vi "MAAP3.vi"(0 "Header Comments":string="This is a C(T) experiment being done in Physics 350.\r\nIt records the decay response of an RC circuit where the capacitance is a strong function of temperature.", 9 "Timing control parameters":T2={"N cycles for averaging"=10, "N points per measurment"=1000, "Measurment time interval"=2e-05} {"Measurment time interval" format="%.2e"}, 11 "error in":errorcluster) -> (3 "Proceed":bool=TRUE, 4 "data file path out":path, 6 "Temp Array":dbl[](array[numeric])=[30.0, 40.0, 50.0, 60.0, 70.0, 80.0], 10 "Timing Control Parameters out":T2={"N cycles for averaging"=10, "N points per measurment"=1000, "Measurment time interval"=2e-05} {"Measurment time interval" format="%.2e"}, 14 "Auto Launch Data Viewer at End":bool=TRUE)   [LabVIEW 2016]
doc: "This vi opens a file from the path input and reads a text header then build temp control and time control parameters. These parametars can be modified manually and then an array of temperatures will be created.\n\nMuhannad Alghamdi\nProject 3\nCSUSB Physics 350"
uses:
  typedefs/time_control_params.ctl
  typedefs/temp_control_params.ctl
panel:
  out "error out":errorcluster
  in  "Temp control parameters":T1={"Start Temp"=30.0, "Temp Step"=10.0, "End Temp"=80.0} {"End Temp" format="%.2f"; "Temp Step" format="%.2f"; "Start Temp" format="%.2f"}
  in  "Reload parameters":bool
  in  "Exit":bool
  in  "Create file and proceed":bool
  out "File Header":string="This is a C(T) experiment being done in Physics 350.\r\nIt records the decay response of an RC circuit where the capacitance is a strong function of temperature.\n\n2/16/2017\n12:19 PM\n\nStart temp = 30.000000\nTemp step = 10.000000\nEnd temp = 80.000000\nNum temps = 6\nNum avg cycles = 10\nNum points per meas = 1000\nMeas time interval = 2.000000E-5\n\n<data below>\n\n"
  out "N temps":i32=6
  in  "Auto Launch Data Viewer at End":bool=TRUE
  # "P350 C(T) Experimental Initialization"
  # "Muhanad Alghamdi\nProject 3\nCSUSB Physics 350"
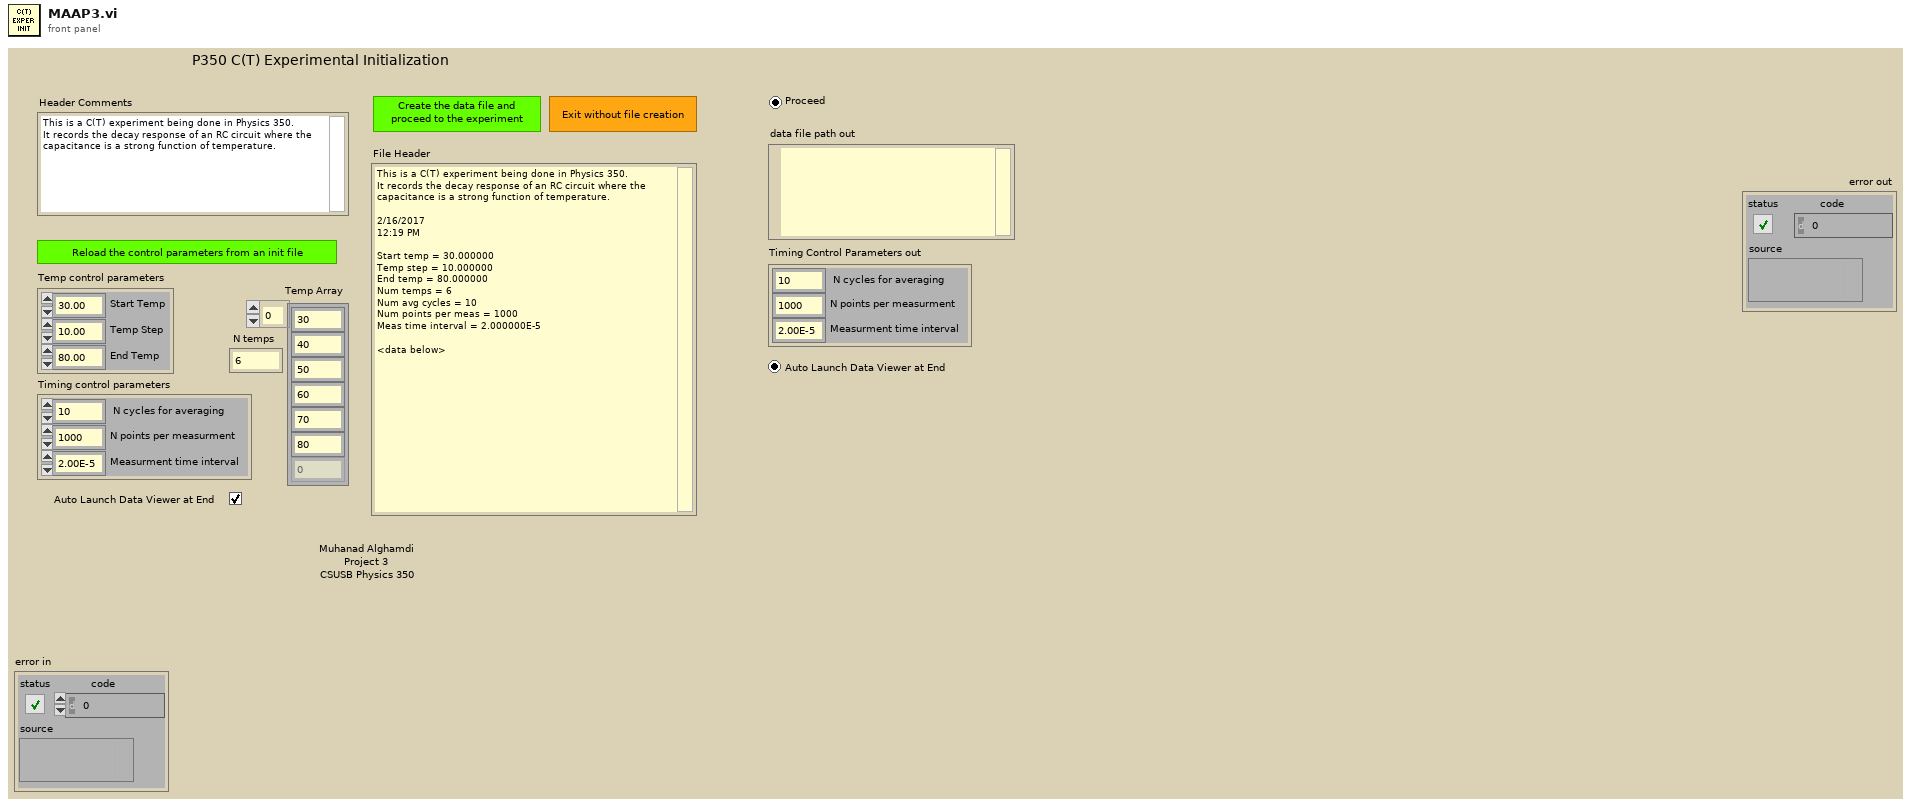
[diagram p1: front panel]
types:
  T1 = typedef "temp_control_params.ctl" = cluster{"Start Temp":dbl, "Temp Step":dbl, "End Temp":dbl}
  T2 = typedef "time_control_params.ctl" = cluster{"N cycles for averaging":i32, "N points per measurment":i32, "Measurment time interval":dbl}
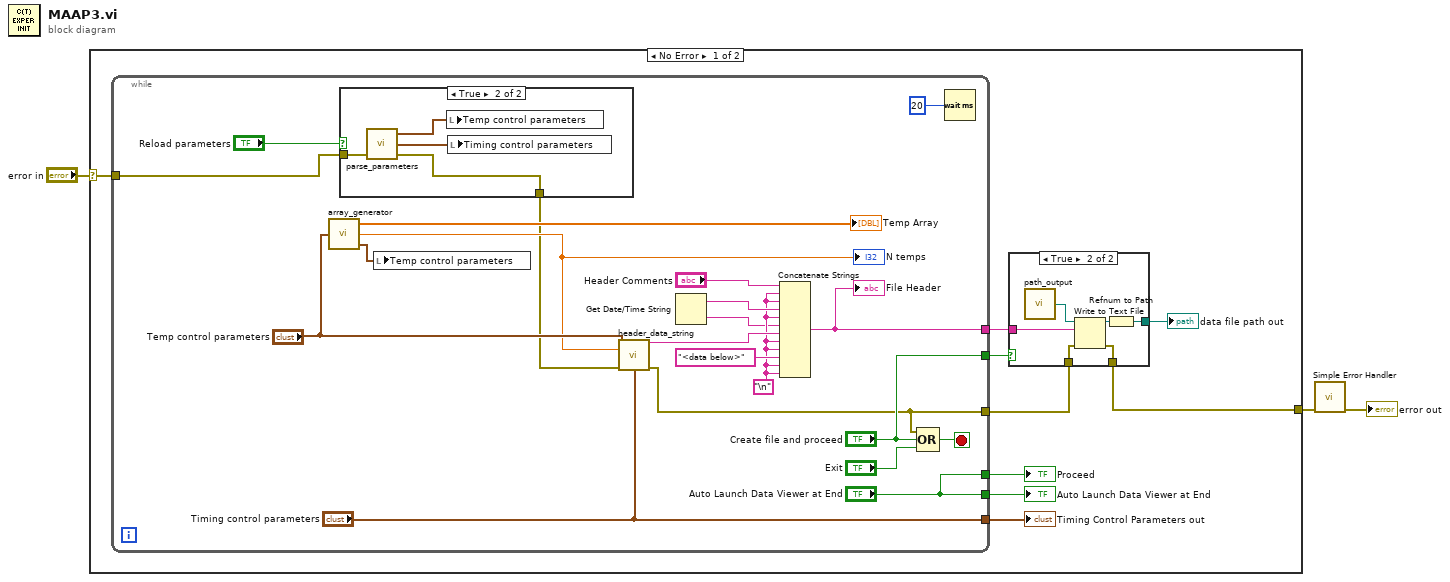
[diagram p0: block diagram]
diagram:
  n1 = case shown="No Error" "error in" {
    selector: "error in" -> [w9 w46]
    tunnel: [w4 w46] -> w1
    frame No Error {
      n2 = while {
        tunnel: ["Timing control parameters"] -> w12
        tunnel: ["Auto Launch Data Viewer at End"] -> w11
        tunnel: ["Auto Launch Data Viewer at End"] -> w10
        tunnel: w9 -> [w24]
        tunnel: ["Create file and proceed"] -> w8
        tunnel: [w22] -> w7
        tunnel: [w21] -> w5
        stop <- w28 stop-if-true
        w33 = "\n"
        n3 = call "array_generator.vi"("Temp control parameters"="Temp control parameters") -> ("Temp array"=→"Temp Array":dbl[], "N temps"=w30:dbl, "Temp control parameters out"=w29:T1)
        "N temps" <- w30
        n4 = case shown="True" "Reload parameters" {
          tunnel: w24 -> [w41 w43]
          tunnel: [w41 w42] -> w25
          frame False {
          }
          frame True {
            n5 = call "parse_parameters.vi"("error in"=w43) -> ("error out"=w42:errorcluster, "Time control parameters"=w45:T2, "Temp control parameters"=w44:T1)  [unwired: 2 in]
            n6 = local write "Temp control parameters"(w44) -> ()
            n7 = local write "Timing control parameters"(w45) -> ()
          }
        }
        n8 = local write "Temp control parameters"(w29) -> ()
        n9 = call "header_data_string.vi"("Temperature Control Parameters"="Temp control parameters", "N temps"=w30, "error in (no error)"=w25, "Timing Control Parameters"="Timing control parameters") -> ("Header string component"=w39:string, "error out"=w21:errorcluster)  [unwired: 10 in]
        n10 = Get Date/Time String() -> (date string=w34:string, time string=w32:string)  [unwired: 3 in]
        n11 = Concatenate Strings("Header Comments", w33, w33, w34, w33, w32, w39, w33, w33, "<data below>", w33, w33) -> (w22:string)
        "File Header" <- w22
        n12 = Compound Arithmetic op=OR(w21, "Create file and proceed", "Exit") -> (w28:bool)
        n13 = Wait (ms)(milliseconds to wait=u32 20) -> ()  [unwired: 1 out]
      }
      "Timing Control Parameters out" <- w12
      "Proceed" <- w11
      "Auto Launch Data Viewer at End" <- w10
      n14 = case shown="True" w8 {
        tunnel: [_ w18] -> w6
        tunnel: w7 -> [_ w17]
        tunnel: w5 -> [w13 w16]
        tunnel: [w13 w15] -> w4
        frame False {
        }
        frame True {
          n15 = call "path_output.vi"() -> ("Path output"=w14:path)  [unwired: 2 in]
          n16 = Write to Text File(file (use dialog)=w14, text=w17, error in=w16) -> (refnum out=w19:refnum<file>, error out=w15:errorcluster)  [unwired: 1 in, 1 out]
          n17 = Refnum to Path(1:w19) -> (0:w18:path)
        }
      }
      "data file path out" <- w6
    }
    frame Error {
    }
  }
  n18 = call <vilib>:"Simple Error Handler.vi"("error in (no error)"=w1) -> ("error out"=→"error out":errorcluster)  [unwired: 4 in, 4 out]
